vi "OpenBkPrecisionInput.vi"(2 "error":errorcluster, 3 "Configuration State":i32, 4 "Configuration Value":dbl, 5 "VISA resource name":refnum<visa-resource-name>) -> (0 "error out 2":errorcluster, 1 "VISA resource name":refnum<visa-resource-name>)   [LabVIEW 2010]
uses:
  Program Files/National Instruments/LabVIEW 2011/instr.lib/BK Precision 85XX Series/BK Precision 85XX Series.lvlib
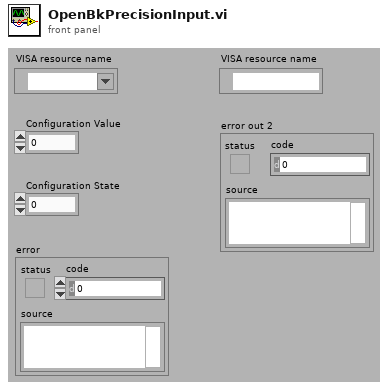
[diagram p1: front panel]
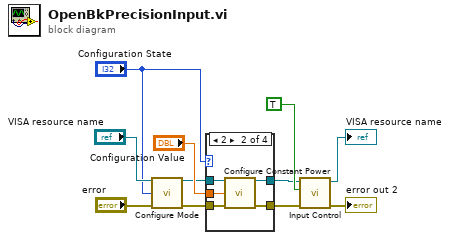
[diagram p0: block diagram]
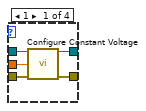
[diagram p2: hidden frame]
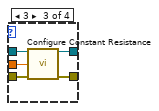
[diagram p3: hidden frame]
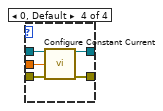
[diagram p4: hidden frame]
diagram:
  n1 = call "Configure Mode.vi"("VISA resource name"="VISA resource name", "Mode of Operation (0:CC)"="Configuration State", "error in (no error)"="error") -> ("VISA resource name out"=w4:refnum<visa-resource-name>, "error out"=w3:errorcluster)  [unwired: 11 in]
  n2 = case shown="2" "Configuration State" {
    tunnel: "Configuration Value" -> [w16 w21 w26 w31]
    tunnel: w4 -> [w15 w20 w25 w29]
    tunnel: w3 -> [w14 w19 w24 w30]
    tunnel: [w13 w18 w23 w28] -> w2
    tunnel: [w12 w17 w22 w27] -> w1
    frame 1 {
      n3 = call "Configure Constant Voltage.vi"("VISA resource name"=w15, "CV Voltage (0)"=w16, "error in (no error)"=w14) -> ("VISA resource name out"=w13:refnum<visa-resource-name>, "error out"=w12:errorcluster)  [unwired: 11 in]
    }
    frame 2 {
      n4 = call "Configure Constant Power.vi"("VISA resource name"=w20, "CW Power (0)"=w21, "error in (no error)"=w19) -> ("VISA resource name out"=w18:refnum<visa-resource-name>, "error out"=w17:errorcluster)  [unwired: 11 in]
    }
    frame 3 {
      n5 = call "Configure Constant Resistance.vi"("VISA resource name"=w25, "CR Resistance (4000)"=w26, "error in (no error)"=w24) -> ("VISA resource name out"=w23:refnum<visa-resource-name>, "error out"=w22:errorcluster)  [unwired: 11 in]
    }
    frame 0, Default {
      n6 = call "Configure Constant Current.vi"("VISA resource name"=w29, "CC Current (0)"=w31, "error in (no error)"=w30) -> ("VISA resource name out"=w28:refnum<visa-resource-name>, "error out"=w27:errorcluster)  [unwired: 11 in]
    }
  }
  n7 = call "Input Control.vi"("error in (no error)"=w1, "Enable Input Terminals (F: Off)"=TRUE, "VISA resource name"=w2) -> ("error out"=→"error out 2":errorcluster, "VISA resource name out"=→"VISA resource name":refnum<visa-resource-name>)  [unwired: 7 in]
